vi "VoltageMeasurement2.vi"(3 "Number of measurements":dbl=2.0, 5 "Measurement wait time (ms)":dbl=300.0, 6 "error in":errorcluster, 8 "Temp Controller address":string="15", 10 "DMM2 GPIB address":string="22", 11 "DMM GPIB address":string="11") -> (0 "Voltage 1 (V)":dbl[](array[numeric])=[-0.320057771, -0.32005326349999996] format="%.6f", 1 "Voltage 2 (V)":dbl[](array[numeric])=[4.000000000000016e-06, 1.2000000000000007e-05, 4.000000000000002e-06, 6.00000000000001e-06, 1.8500000000000002e-05] format="%.6f", 2 "Temperature (C)":dbl[](array[numeric])=[4.000000000000016e-06, 1.2000000000000007e-05, 4.000000000000002e-06, 6.00000000000001e-06, 1.8500000000000002e-05] format="%.6f", 4 "error out":errorcluster)   [LabVIEW 2014]
uses:
  <vilib>/Analysis/baseanly.llb/Mean (DBL).vi
  <vilib>/Analysis/NI_AALBase.lvlib
panel:
  out "V1 average (V)":dbl=-0.32005551725 format="%.4e"
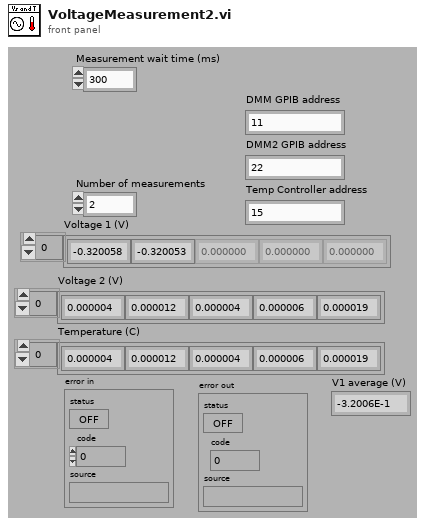
[diagram p1: front panel]
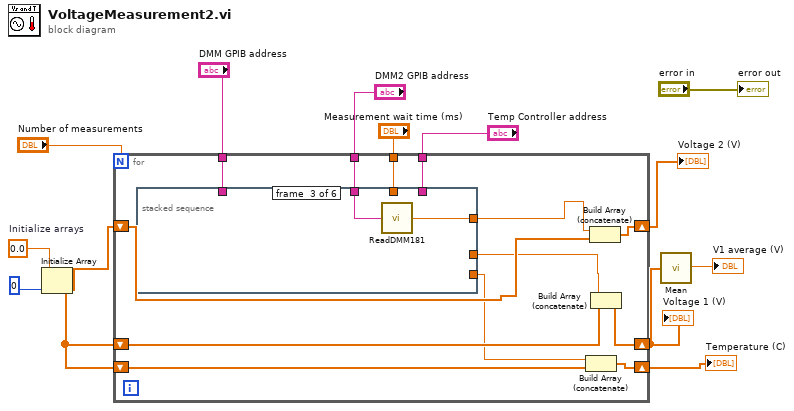
[diagram p0: block diagram]
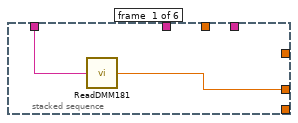
[diagram p2: hidden frame]
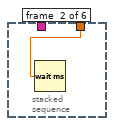
[diagram p3: hidden frame]
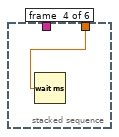
[diagram p4: hidden frame]
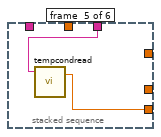
[diagram p5: hidden frame]
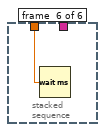
[diagram p6: hidden frame]
diagram:
  w11 = 0.0  # Initialize arrays
  n1 = Initialize Array(w11, 0) -> (w2:dbl[])
  n2 = for {
    N: "Number of measurements" -> [_]
    shift-right: [w23] -> w6
    shift-left: w2 -> [w25]
    tunnel: "DMM GPIB address" -> [w26]
    tunnel: "Measurement wait time (ms)" -> [w24]
    tunnel: "DMM2 GPIB address" -> [w22]
    tunnel: "Temp Controller address" -> [w21]
    shift-right: [w20] -> w3
    shift-left: w2 -> [w19]
    shift-right: [w16] -> w1
    shift-left: w2 -> [w15]
    n3 = stacked-sequence {
      tunnel: w26 -> [w28 _ _ _ _ _]
      tunnel: [w27 _ _ _ _ _] -> w17
      tunnel: w24 -> [_ w29 _ w32 _ w35]
      tunnel: w22 -> [_ _ w31 _ _ _]
      tunnel: w21 -> [_ _ _ _ w34 _]
      tunnel: [_ _ w30 _ _ _] -> w18
      tunnel: [_ _ _ _ w33 _] -> w14
      frame #0 {
        n4 = call "ReadDMM181.vi"("DMM GPIB Address"=w28) -> ("DMM read (V)"=w27:dbl)
      }
      frame #1 {
        n5 = Wait (ms)(milliseconds to wait=w29) -> ()  [unwired: 1 out]
      }
      frame #2 {
        n6 = call "ReadDMM181.vi"("DMM GPIB Address"=w31) -> ("DMM read (V)"=w30:dbl)
      }
      frame #3 {
        n7 = Wait (ms)(milliseconds to wait=w32) -> ()  [unwired: 1 out]
      }
      frame #4 {
        n8 = call "tempcondread.vi"("GPIB Address"=w34) -> ("Temperature"=w33:dbl)  [unwired: 2 in, 1 out]
      }
      frame #5 {
        n9 = Wait (ms)(milliseconds to wait=w35) -> ()  [unwired: 1 out]
      }
    }
    n10 = Build Array (concatenate)(w14, w15) -> (w16:dbl[])
    n11 = Build Array (concatenate)(w18, w19) -> (w20:dbl[])
    n12 = Build Array (concatenate)(w17, w25) -> (w23:dbl[])
  }
  "Voltage 1 (V)" <- w6
  "Voltage 2 (V)" <- w3
  "Temperature (C)" <- w1
  n13 = call-poly <vilib>:"Mean.vi"("X"=w6) -> ("mean"=→"V1 average (V)":dbl)  [unwired: 1 out]
  "error out" <- "error in"
